vi "TCP-IP Mgr.Disconnect.vi"(8 "error in":errorcluster, 11 "Q Name":string="TCP-IP Mgr") -> (0 "error out":errorcluster)   [LabVIEW 2024, in "EQMF.lvlib" / "TCP-IP.lvlib"]
uses:
  TCP-IP.lvlib
  Queues/Queue Utils.lvlib
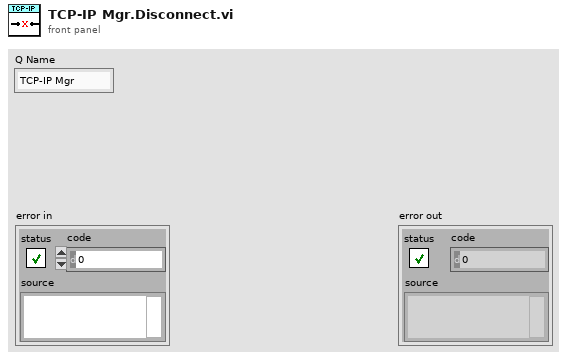
[diagram p1: front panel]
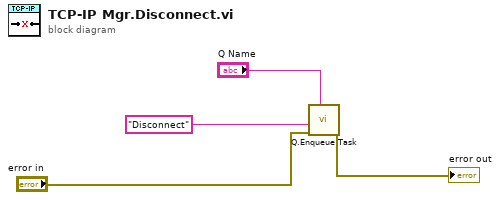
[diagram p0: block diagram]
diagram:
  n1 = call "Q.Enqueue Task.vi"("Q Name"="Q Name", "Error In"="error in", "Task Name"="Disconnect") -> ("error out"=→"error out":errorcluster)  [unwired: 7 in, 1 out]
